vi "Set Width.vi"(8 "Error In":errorcluster, 10 "Width":u32, 11 "Pixel In":refnum<class "Graph.lvclass">) -> (0 "Error Out":errorcluster, 3 "Pixel Out":refnum<class "Graph.lvclass">)   [LabVIEW 2019, in "Graph.lvclass"]
uses:
  Graph.lvclass
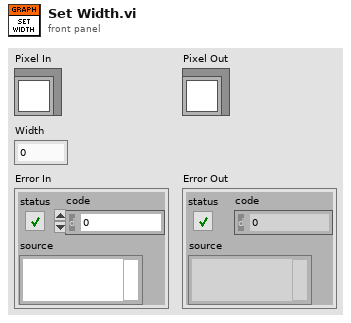
[diagram p1: front panel]
types:
  T1 = typedef "Graph.lvclass/Data.ctl" = cluster{"Height":u32, "Width":u32, "Range":T2, "Data":i32[], "Fill To":T3}
  T2 = typedef "Graph.lvclass/Range.ctl" = cluster{"Maximum":i32, "Minimum":i32}
  T3 = typedef "Graph.lvclass/Fill To.ctl" = enum16{"None", "Zero", "Inf", "-Inf"}
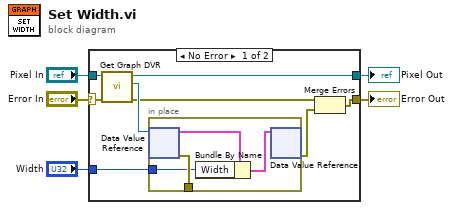
[diagram p0: block diagram]
diagram:
  n1 = case shown="No Error" "Error In" {
    selector: "Error In" -> [w10 w18]
    tunnel: [w12 w18] -> w4
    tunnel: [w7 w19] -> w2
    tunnel: "Pixel In" -> [w9 w19]
    tunnel: "Width" -> [w11 _]
    frame No Error {
      n2 = call "Get Graph DVR.vi"("Error In"=w10, "Graph In"=w9) -> ("Error Out"=w6:errorcluster, "DVR"=w8:refnum<data-value>, "Graph Out"=w7:refnum<class "Graph.lvclass">)  [unwired: 7 in]
      n3 = in-place {
        in-place-border: [w17] -> _
        in-place-border: w11 -> [w14]
        n4 = in-place-dvr #1(w8) -> (w16:T1, w17:errorcluster)
        n5 = Bundle By Name(cluster=w16, "Width"=w14) -> (w15:T1)
        n6 = in-place-dvr #1(w15) -> (w13:errorcluster)  [unwired: 1 out]
      }
      n7 = Merge Errors(w6, w13) -> (w12:errorcluster)
    }
    frame Error {
    }
  }
  "Pixel Out" <- w2
  "Error Out" <- w4
